vi "Test_Localization_Algorithm-1.vi"() -> ()   [LabVIEW 2020]
panel:
  in  "[IN] Method":i32(ring) items=["clustering", "entropy", "metric", "moments", "inter-class variance"]
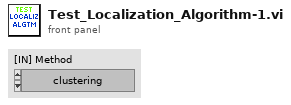
[diagram p1: front panel]
types:
  T1 = typedef "Image Type" = u32
  T2 = typedef "IMAQ Image.ctl" = refnum<image>
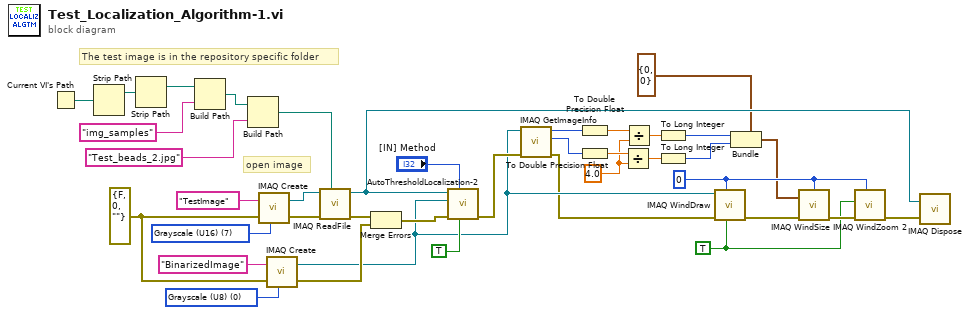
[diagram p0: block diagram]
diagram:
  w6 = 4.0 ("y")
  w5 = TRUE ("Scrollbars? (N)")
  w31 = T1 0 items=["Grayscale (U8)", "Grayscale (I16)", "Grayscale (SGL)", "Complex (CSG)", "RGB (U32)", "HSL (U32)", "RGB (U64)", "Grayscale (U16)"] ("Image Type")
  w21 = 0 ("Window Number (0...15)")
  w35 = T1 7 items=["Grayscale (U8)", "Grayscale (I16)", "Grayscale (SGL)", "Complex (CSG)", "RGB (U32)", "HSL (U32)", "RGB (U64)", "Grayscale (U16)"] ("Image Type")
  w30 = errorcluster {"status"=FALSE, "code"=0, "source"=""} ("error in (no error)")
  # "open image"
  # "The test image is in the repository specific folder"
  n1 = Current VI's Path() -> (path=w39:path)
  n2 = Strip Path(path=w39) -> (stripped path=w4:path)  [unwired: 1 out]
  n3 = Strip Path(path=w4) -> (stripped path=w3:path)  [unwired: 1 out]
  n4 = Build Path(base path=w3, name or relative path="img_samples") -> (appended path=w1:path)
  n5 = Build Path(base path=w1, name or relative path="Test_beads_2.jpg") -> (appended path=w37:path)
  n6 = call "IMAQ Create"("Image Name"="TestImage", "Image Type"=w35, "error in (no error)"=w30) -> ("New Image"=w33:T2, "error out"=w34:errorcluster)  [unwired: 2 in]
  n7 = call "IMAQ Create"("Image Name"="BinarizedImage", "Image Type"=w31, "error in (no error)"=w30) -> ("New Image"=w18:T2, "error out"=w28:errorcluster)  [unwired: 2 in]
  n8 = call "IMAQ ReadFile"("File Path"=w37, "error in (no error)"=w34, "Image"=w33) -> ("error out"=w29:errorcluster, "Image Out"=w24:T2)  [unwired: 4 in, 3 out]
  n9 = Merge Errors(w29, w28) -> (w27:errorcluster)
  n10 = call "AutoThresholdLocalization-2.vi"("[IN] Autothreshold Images \nInstead Of Generated U8"=TRUE ("[IN] Autothreshold Images \nInstead Of Generated U8"), "[IN] Method"="[IN] Method", "error IN"=w27, "[IN] Binarized Image"=w18, "[IN] Source Image"=w24) -> ("error OUT"=w19:errorcluster)  [unwired: 5 in, 1 out]
  n11 = call "IMAQ GetImageInfo"("error in (no error)"=w19, "Image"=w18) -> ("error out"=w10:errorcluster, "Y Resolution"=w13:i32, "X Resolution"=w16:i32)  [unwired: 2 in, 5 out]
  n12 = To Double Precision Float(number=w16) -> (double precision float=w15:dbl)
  n13 = To Double Precision Float(number=w13) -> (double precision float=w12:dbl)
  n14 = Divide(x=w12, y=w6) -> (x/y=w11:dbl)
  n15 = Divide(x=w15, y=w6) -> (x/y=w14:dbl)
  n16 = To Long Integer(number=w14) -> (32bit integer=w8:i32)
  n17 = To Long Integer(number=w11) -> (32bit integer=w7:i32)
  n18 = call "IMAQ WindDraw"("Resize to Image Size? (Y)"=w5, "Window Number (0...15)"=w21, "error in (no error)"=w10, "Image"=w18) -> ("error out"=w22:errorcluster)  [unwired: 6 in, 1 out]
  n19 = Bundle(cluster=cluster{"Width":i32, "Height":i32} {"Width"=0, "Height"=0} ("Width & Height"), "Width"=w8, "Height"=w7) -> (w9:cluster{"Width":i32, "Height":i32})
  n20 = call "IMAQ WindSize"("error in (no error)"=w22, "Width & Height"=w9, "Window Number"=w21) -> ("error out"=w20:errorcluster)  [unwired: 3 in, 2 out]
  n21 = call "IMAQ WindZoom 2"("Window Number (0...15)"=w21, "error in (no error)"=w20, "Zoom to Fit? (False)"=w5) -> ("error out"=w23:errorcluster)  [unwired: 5 in, 3 out]
  n22 = call "IMAQ Dispose"("Image"=w24, "error in (no error)"=w23) -> ()  [unwired: 4 in, 1 out]
